vi "Inline Image.vi"(5 "Image ID (\"\")":string, 6 "Image Size":cluster{"width":i32, "height":i32}, 7 "Image (Empty Picture)":picture) -> (3 "HTML out":string)   [LabVIEW 2011]
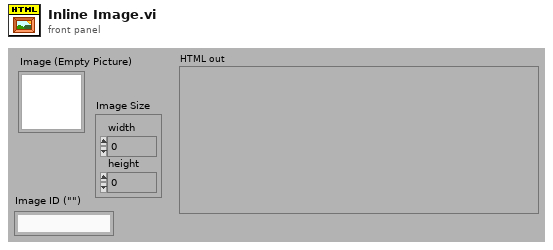
[diagram p1: front panel]
types:
  T1 = cluster{"left":i16, "top":i16, "right":i16, "bottom":i16}
  T2 = typedef "imagedata.ctl" = cluster{"image type":i32, "image depth":i32, "image":u8[], "mask":u8[], "colors":u32[], "Rectangle":cluster{"left":i16, "top":i16, "right":i16, "bottom":i16}}
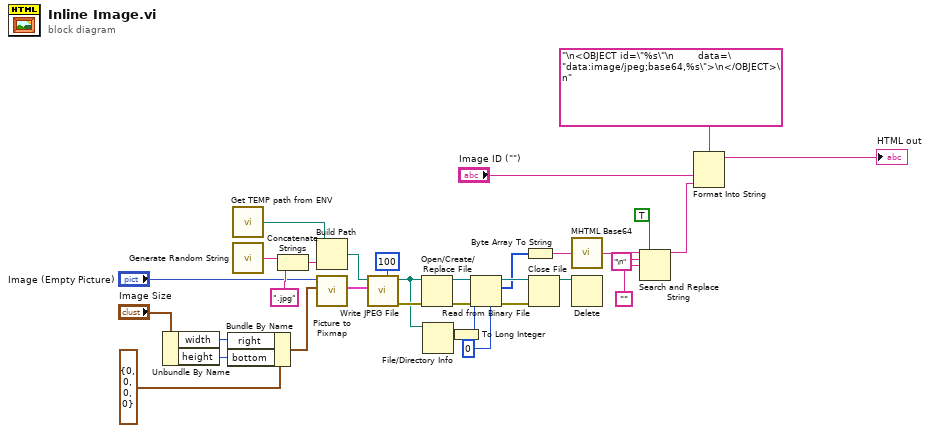
[diagram p0: block diagram]
diagram:
  n1 = Unbundle By Name("Image Size") -> ("width"=w9:i32, "height"=w8:i32)
  n2 = Bundle By Name(cluster=T1 {"left"=0, "top"=0, "right"=0, "bottom"=0} ("rect"), "right"=w9, "bottom"=w8) -> (w11:T1)
  n3 = call "Get TEMP path from ENV.vi"() -> ("TEMP Path"=w31:path)  [unwired: 5 out]
  n4 = call "Generate Random String.vi"() -> ("Output String"=w30:string)  [unwired: 1 in, 4 out]
  n5 = Concatenate Strings(w30, ".jpg") -> (w28:string)
  n6 = Build Path(base path=w31, name or relative path=w28) -> (appended path=w27:path)
  n7 = call <vilib>:"Picture to Pixmap.vi"("rect"=w11, "picture"="Image (Empty Picture)") -> ("image data"=w23:T2)  [unwired: 2 in, 7 out]
  n8 = call <vilib>:"Write JPEG File.vi"("quality (80)"=100 ("compression (default)"), "image data"=w23, "path to JPEG file"=w27) -> ("error out"=w25:errorcluster, "path"=w17:path)  [unwired: 1 in, 6 out]
  n9 = Open/Create/Replace File(file path (use dialog)=w17, error in=w25) -> (refnum out=w22:refnum<file>, error out=w21:errorcluster)  [unwired: 5 out]
  n10 = File/Directory Info(path=w17) -> (size=w1:i64)  [unwired: 1 in, 6 out]
  n11 = To Long Integer(number=w1) -> (32bit integer=w16:i32)
  n12 = Read from Binary File(5:u8 0, 8:w21, 10:w16, 11:w22) -> (0:w19:errorcluster, 2:w13:u8[], 3:w20:refnum<file>)  [unwired: 3 out]
  n13 = Byte Array To String(unsigned byte array=w13) -> (string=w14:string)
  n14 = Close File(refnum=w20, error in=w19) -> (path=w18:path)  [unwired: 1 out]
  n15 = call "MHTML Base64.vi"("Binary String"=w14) -> ("String (Base64)"=w5:string)  [unwired: 14 out]
  n16 = Delete(path (use dialog)=w18) -> ()  [unwired: 1 in, 6 out]
  n17 = Search and Replace String(replace all?=TRUE, input string=w5, search string="\n", replace string="") -> (result string=w4:string)  [unwired: 1 in, 6 out]
  n18 = Format Into String(format string="\n<OBJECT id=\"%s\"\n        data=\"data:image/jpeg;base64,%s\">\n</OBJECT>\n", "Image ID (\"\")", w4) -> (resulting string=→"HTML out":string)  [unwired: 2 in, 1 out]
